vi "CaracterizacionDiodo.vi"(0 "Voltaje inicial:":dbl, 1 "Voltaje":T1, 2 "Enum":enum16{"Alim1", "Alim2"}(ring), 5 "Paso":dbl, 9 "Voltaje final:":dbl, 11 "Voltaje  2":T1, 12 "Corriente":T1) -> (3 "Voltaje":T1, 4 "Voltaje":dbl[](array[numeric]), 6 "Corriente":dbl[](array[numeric]), 10 "Error?":bool, 14 "Corriente":T1)   [LabVIEW 2017]
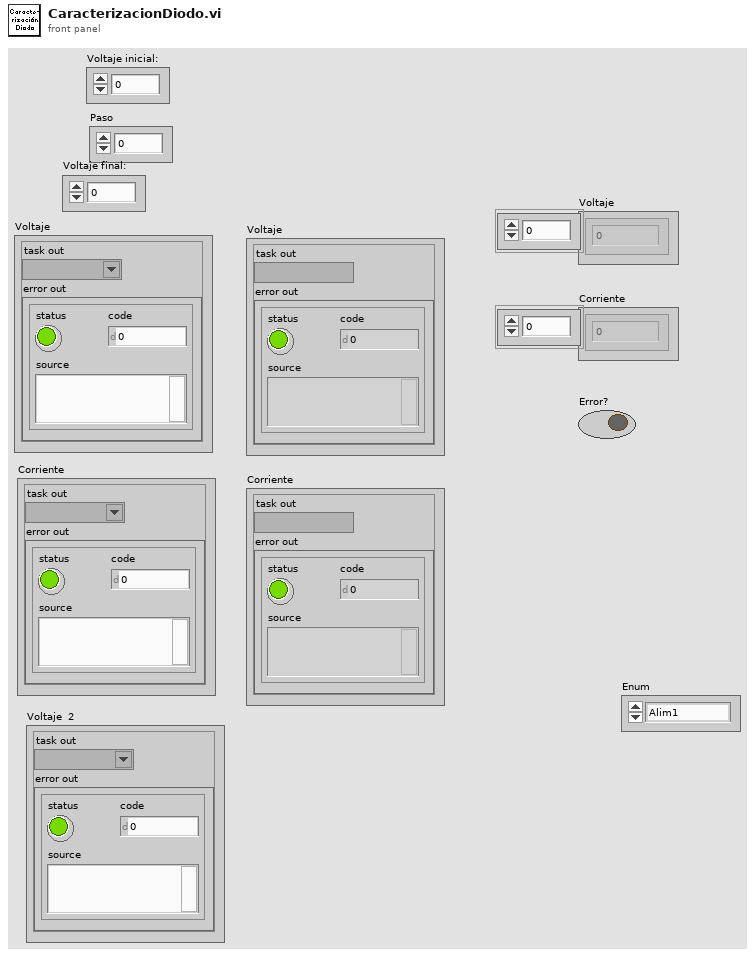
[diagram p1: front panel]
types:
  T1 = cluster{"task out":refnum<k21>, "error out":errorcluster}
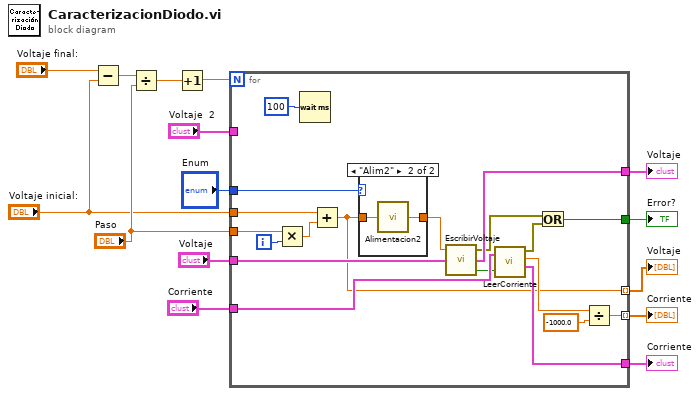
[diagram p0: block diagram]
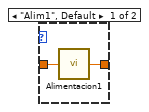
[diagram p2: hidden frame]
diagram:
  n1 = Subtract(x="Voltaje final:", y="Voltaje inicial:") -> (x-y=w9:dbl)
  n2 = Divide(x=w9, y="Paso") -> (x/y=w5:dbl)
  n3 = Increment(x=w5) -> (x+1=w3:dbl)
  n4 = for {
    N: w3 -> [_]
    tunnel: "Paso" -> [w34]
    tunnel: [w24] -> w15 mode=indexing
    tunnel: "Voltaje inicial:" -> [w32]
    tunnel: [w30] -> w13
    tunnel: "Voltaje  2" -> [_]
    tunnel: "Voltaje" -> [w28]
    tunnel: [w27] -> w14
    tunnel: "Corriente" -> [w22]
    tunnel: [w20] -> w12
    tunnel: [w18] -> w2 mode=indexing
    tunnel: "Enum" -> [w16]
    i -> [w33]
    n5 = Multiply(x=w34, y=w33) -> (x*y=w31:dbl)
    n6 = Wait (ms)(milliseconds to wait=u32 100) -> ()  [unwired: 1 out]
    n7 = Add(x=w32, y=w31) -> (x+y=w18:dbl)
    n8 = case shown="\"Alim2\"" w16 {
      tunnel: [w35 w37] -> w19
      tunnel: w18 -> [w36 w38]
      frame "Alim1", Default {
        n9 = call "Alimentacion1.vi"("VoltajeDeseado"=w36) -> ("Numeric Indicator"=w35:dbl)
      }
      frame "Alim2" {
        n10 = call "Alimentacion2.vi"("VoltajeDeseado"=w38) -> ("Numeric Indicator"=w37:dbl)
      }
    }
    n11 = call "EscribirVoltaje.vi"("cluster"=w28, "data"=w19) -> ("Boolean 2"=w21:bool, "Cluster"=w27:T1, "error out"=w26:errorcluster)  [unwired: 1 in]
    n12 = call "LeerCorriente.vi"("output cluster"=w22, "Boolean"=w21) -> ("error out"=w23:errorcluster, "data"=w29:dbl, "Cluster"=w20:T1)  [unwired: 1 out]
    n13 = Or(x=w26, y=w23) -> (x .or. y?=w30:bool)
    n14 = Divide(x=w29, y=-1000.0) -> (x/y=w24:dbl)
  }
  "Corriente" <- w15
  "Voltaje" <- w2
  "Voltaje" <- w14
  "Error?" <- w13
  "Corriente" <- w12
